vi "Set Module Vacuum.vi"(6 "On/Off":bool, 8 "error in":errorcluster, 9 "Slot Number":i32, 10 "Chuck Number":i32, 11 "Gantry in":refnum<class "Gantry Class.lvclass">) -> (0 "error out":errorcluster, 3 "Gantry out":refnum<class "Gantry Class.lvclass">)   [LabVIEW 2017, in "Gantry Class.lvclass"]
uses:
  Gantry Class.lvclass
  WorkTable Class/WorkTable Class.lvclass
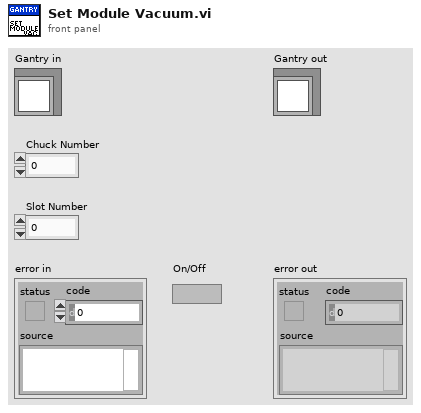
[diagram p1: front panel]
types:
  T1 = typedef "Worktable_Module Slot.ctl" = cluster{"Slot State":enum16{"Empty", "Bare HDI", "Unglued", "Stamped", "PartOnTop", "Weighted", "Unpotted", "Potted"}, "BBM Type":enum16{"None", "BBM", "GlassSlide"}, "HDI Type":enum16{"None", "HDI", "Polyimide"}, "Vacuum Channel":u8, "Location/Orientation BBM":T2, "Location/Orientation HDI":T2, "S/N":string}
  T2 = typedef "Position_Orientation.ctl" = cluster{"Center":refnum<class "Vec3d Class.lvclass">, "Orientation":refnum<class "Orient3d Class.lvclass">}
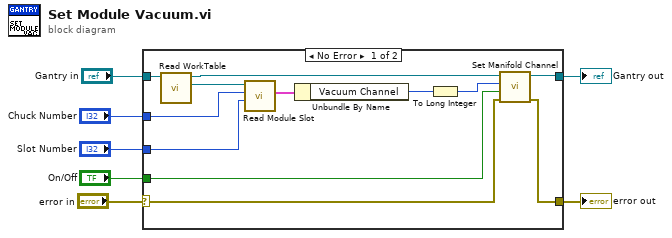
[diagram p0: block diagram]
diagram:
  n1 = case shown="No Error" "error in" {
    selector: "error in" -> [w8 w21]
    tunnel: [w13 w21] -> w6
    tunnel: [w14 w20] -> w4
    tunnel: "Gantry in" -> [w19 w20]
    tunnel: "Chuck Number" -> [w12 _]
    tunnel: "Slot Number" -> [w11 _]
    tunnel: "On/Off" -> [w16 _]
    frame No Error {
      n2 = call-dynamic "Read WorkTable.vi"("Gantry Class in"=w19) -> ("WorkTable Class.lvclass"=w18:refnum<class "WorkTable Class.lvclass">, "Gantry Class out"=w15:refnum<class "Gantry Class.lvclass">)  [unwired: 8 in, 1 out]
      n3 = call-dynamic "Read Module Slot.vi"("slot"=w11, "chuck"=w12, "WorkTable in"=w18) -> ("Module Slot"=w17:T1)  [unwired: 6 in, 2 out]
      n4 = Unbundle By Name(w17) -> ("Vacuum Channel"=w10:u8)
      n5 = To Long Integer(number=w10) -> (32bit integer=w9:i32)
      n6 = call-dynamic "Set Manifold Channel.vi"("error in"=w8, "On/Off"=w16, "Manifold Channel"=w9, "Gantry in"=w15) -> ("error out"=w13:errorcluster, "Gantry out"=w14:refnum<class "Gantry Class.lvclass">)  [unwired: 6 in]
    }
    frame Error {
    }
  }
  "error out" <- w6
  "Gantry out" <- w4
